vi "Fetch Waveform (Voltage).vi"(0 "VISA resource name":refnum<visa-resource-name>, 11 "error in (no error)":errorcluster) -> (4 "VISA resource name out":refnum<visa-resource-name>, 6 "Waveform (V)":waveform(dbl), 15 "error out":errorcluster)   [LabVIEW 2012, in "NH Research Regenerative Test Series.lvlib"]
doc: "Return a waveform containing the instantaneous input voltage in Volts. Query Number of Samples is called internally to read how many samples are available to read from the instruments buffer. Note that the initial time returned will be 0 (unused) since this vi does not initiate a measurement. Because it only retrieve samples from the instrument's buffer, it does not have knowledge if the time when the measurement was initiated.\n\nWaveforms are captured with every initiated measurement based on the Set Aperture Length.vi and Set Number of Samples.vi commands. A measurement must be initiated first using a Read command or calling Initiate Measurement.vi."
uses:
  <instrlib>/NH Research Regenerative Test Series/NH Research Regenerative Test Series.lvlib
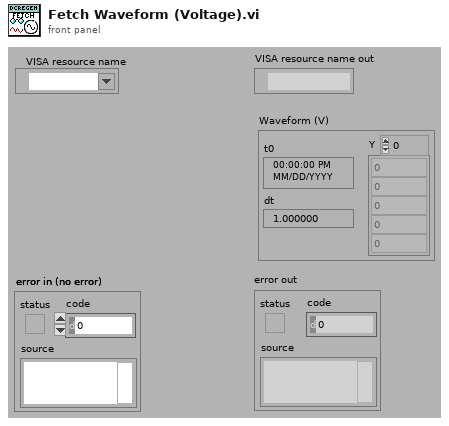
[diagram p1: front panel]
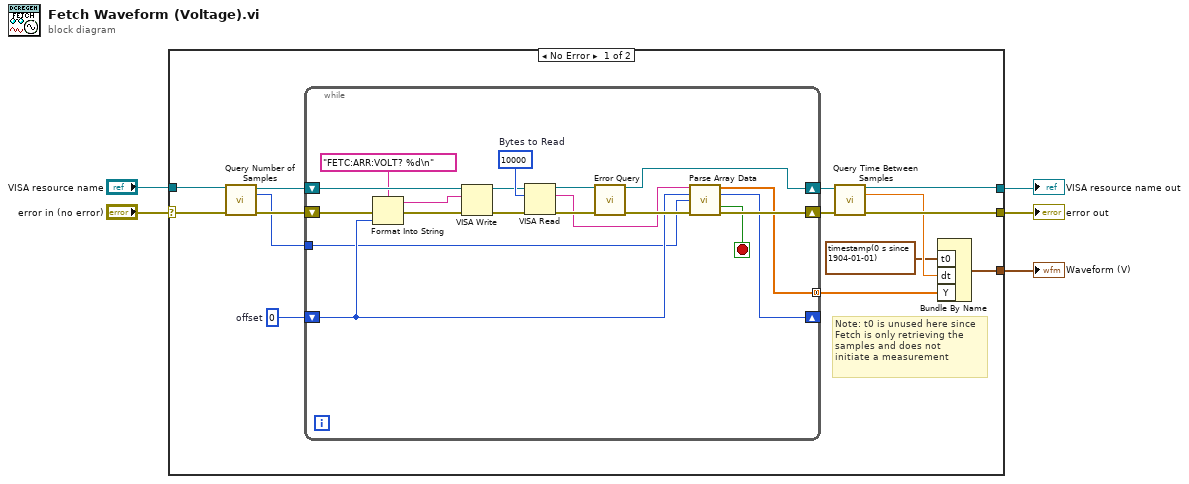
[diagram p0: block diagram]
diagram:
  n1 = case shown="No Error" "error in (no error)" {
    selector: "error in (no error)" -> [w18 w40]
    tunnel: [w10 w40] -> w4
    tunnel: [w7 w39] -> w2
    tunnel: "VISA resource name" -> [w17 w39]
    tunnel: [w8 _] -> w1
    frame No Error {
      w19 = 0  # offset
      # "Note: t0 is unused here since\nFetch is only retrieving the\nsamples and does not\ninitiate a measurement"
      n2 = call <instrlib>:"Query Number of Samples.vi"("VISA resource name"=w17, "error in (no error)"=w18) -> ("VISA resource name out"=w16:refnum<visa-resource-name>, "Number of Samples"=w14:u32, "error out"=w15:errorcluster)  [unwired: 11 in]
      n3 = while {
        shift-right: [w27] -> w12
        shift-left: w15 -> [w31]
        shift-right: [w20] -> w13
        shift-left: w16 -> [w35]
        tunnel: [w22] -> w11 mode=concatenating
        shift-right: [w23] -> _
        shift-left: w19 -> [w25]
        tunnel: w14 -> [w24]
        stop <- w21 stop-if-true
        w38 = u32 10000  # Bytes to Read
        n4 = Format Into String(format string="FETC:ARR:VOLT? %d\n", error in=w31, w25) -> (resulting string=w29:string, error out=w30:errorcluster)  [unwired: 1 in]
        n5 = VISA Write(VISA resource name=w35, write buffer=w29, error in (no error)=w30) -> (VISA resource name out=w36:refnum<visa-resource-name>, error out=w37:errorcluster)  [unwired: 1 out]
        n6 = VISA Read(VISA resource name=w36, byte count=w38, error in (no error)=w37) -> (VISA resource name out=w34:refnum<visa-resource-name>, read buffer=w26:string, error out=w33:errorcluster)  [unwired: 1 out]
        n7 = call <instrlib>:"Error Query.vi"("VISA resource name"=w34, "error in (no error)"=w33) -> ("VISA resource name out"=w20:refnum<visa-resource-name>, "error out"=w28:errorcluster)  [unwired: 10 in, 2 out]
        n8 = call <instrlib>:"Parse Array Data.vi"("Samples String"=w26, "Current Index"=w25, "Number of Samples"=w24, "error in (no error)"=w28) -> ("Samples"=w22:dbl[], "Next Index"=w23:i32, "Stop Reading Samples"=w21:bool, "error out"=w27:errorcluster)  [unwired: 8 in]
      }
      n9 = call <instrlib>:"Query Time Between Samples.vi"("VISA resource name"=w13, "error in (no error)"=w12) -> ("VISA resource name out"=w7:refnum<visa-resource-name>, "Time Interval (s)"=w9:dbl, "error out"=w10:errorcluster)  [unwired: 11 in]
      n10 = Bundle By Name("t0"=timestamp(0 s since 1904-01-01), "dt"=w9, "Y"=w11) -> (w8:waveform(dbl))  [unwired: 1 in]
    }
    frame Error {
    }
  }
  "error out" <- w4
  "VISA resource name out" <- w2
  "Waveform (V)" <- w1
